vi "Translation3d_NearestTo.vi"(9 "Other Translation3d":T1[](array[typedef]) {"Z" format="%14.3f"; "Y" format="%14.3f"; "X" format="%14.3f"}, 11 "In Translation3d":T1 {"Z" format="%14.3f"; "Y" format="%14.3f"; "X" format="%14.3f"}) -> (1 "Found":bool, 3 "Nearest Translation3d":T1 {"Z" format="%14.3f"; "Y" format="%14.3f"; "X" format="%14.3f"})   [LabVIEW 2019, in "Trajectory_Library.lvlib"]
doc: "Returns the inverse of the current translation. This is equivalent to negating all components of the translation.\n \nParameters:\n - In Translation3d - This translation3d data structure\n\nResult:\n - Out Translation3d - The inverse of the current translation."
uses:
  TypeDef/TRANSLATION3D.ctl
  Trajectory_Library.lvlib
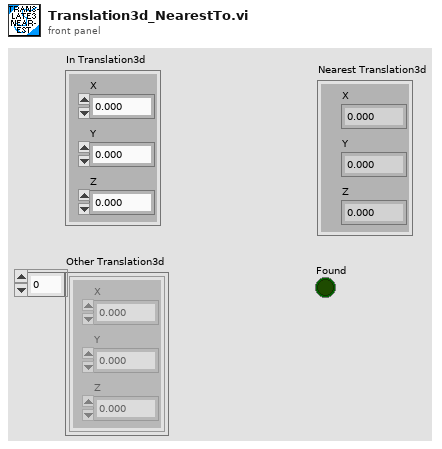
[diagram p1: front panel]
types:
  T1 = typedef "Trajectory_Library.lvlib/TRANSLATION3D.ctl" = cluster{"X":dbl, "Y":dbl, "Z":dbl}
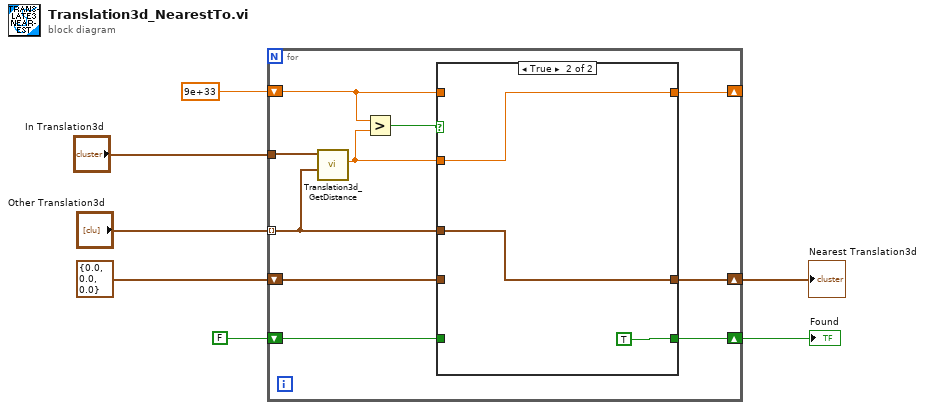
[diagram p0: block diagram]
diagram:
  n1 = for {
    shift-right: [w14] -> _
    shift-left: 9e+33 -> [w10]
    tunnel: "In Translation3d" -> [w17]
    tunnel: "Other Translation3d" -> [w15] mode=indexing
    shift-right: [w11] -> w1
    shift-left: FALSE -> [w8]
    shift-right: [w12] -> w2
    shift-left: T1 {"X"=0.0, "Y"=0.0, "Z"=0.0} ("Other Translation3d") -> [w9]
    n2 = call "Translation3d_GetDistance.vi"("other Translation3d"=w15, "In Translation3d"=w17) -> ("Distance"=w13:dbl)  [unwired: 9 in]
    n3 = Greater?(x=w10, y=w13) -> (0:w16:bool)
    n4 = case shown="True" w16 {
      tunnel: w15 -> [_ w22]
      tunnel: [w20 w23] -> w14
      tunnel: w13 -> [_ w23]
      tunnel: [w19 w22] -> w12
      tunnel: [w18 TRUE] -> w11
      tunnel: w10 -> [w20 _]
      tunnel: w9 -> [w19 _]
      tunnel: w8 -> [w18 _]
      frame False {
      }
      frame True {
      }
    }
  }
  "Nearest Translation3d" <- w2
  "Found" <- w1
